vi "Notif 1.vi"() -> (3 "String":string="Insufficient File Path")   [LabVIEW 2023]
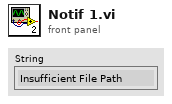
[diagram p1: front panel]
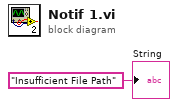
[diagram p0: block diagram]
diagram:
  "String" <- "Insufficient File Path"
